vi "Car wash.vi"() -> ()   [LabVIEW 2019]
uses:
  <vilib>/regexp/Match Regular Expression.xnode
panel:
  out "STATE":string
  out "Vehicle Out Of Position":bool
  out "Air Dry LED":bool
  out "Clear Water Rinse":bool
  out "Main High Pressure Wash":bool
  out "Soap Application":bool
  out "Under Body Wash":bool
  out "Time Left (Sec)":dbl
  in  "Air Dry":bool
  in  "Main Wash":bool
  in  "Under Body":bool
  out "STOP":bool
  in  "stop":bool
  out "ECONOMY":bool
  out "DELUXE":bool
  in  "ECONOMY WASH":bool
  in  "DELUXE WASH":bool
  # "Car Wash Indicators"
  # "Under Body Wash"
  # "Soap Application"
  # "Main High Pressure Wash"
  # "Under Body Wash Position Switch"
  # "Clear Water Rinse"
  # "Main Wash Position Switch"
  # "Air Dry"
  # "Air Dry Position Switch"
  # "Vehicle Out of Position"
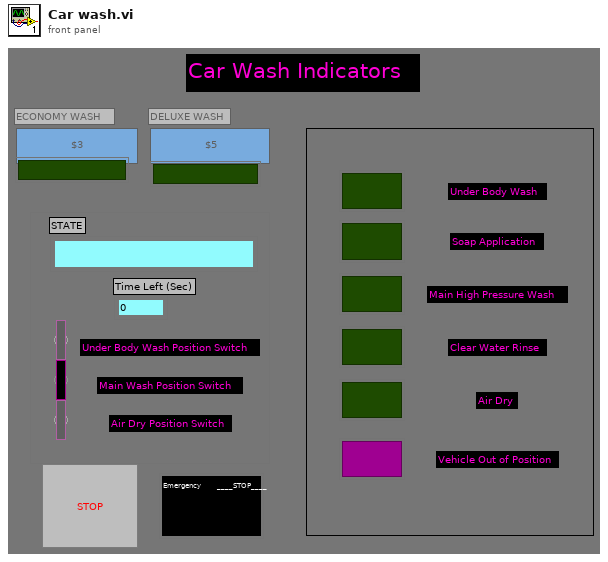
[diagram p1: front panel]
types:
  T1 = enum16{"Station", "Under Body", "Main Body", "Air Dry", "Report", "Stop"}
  T2 = enum8{"Enabled", "Disabled", "Disabled and Grayed Out"}
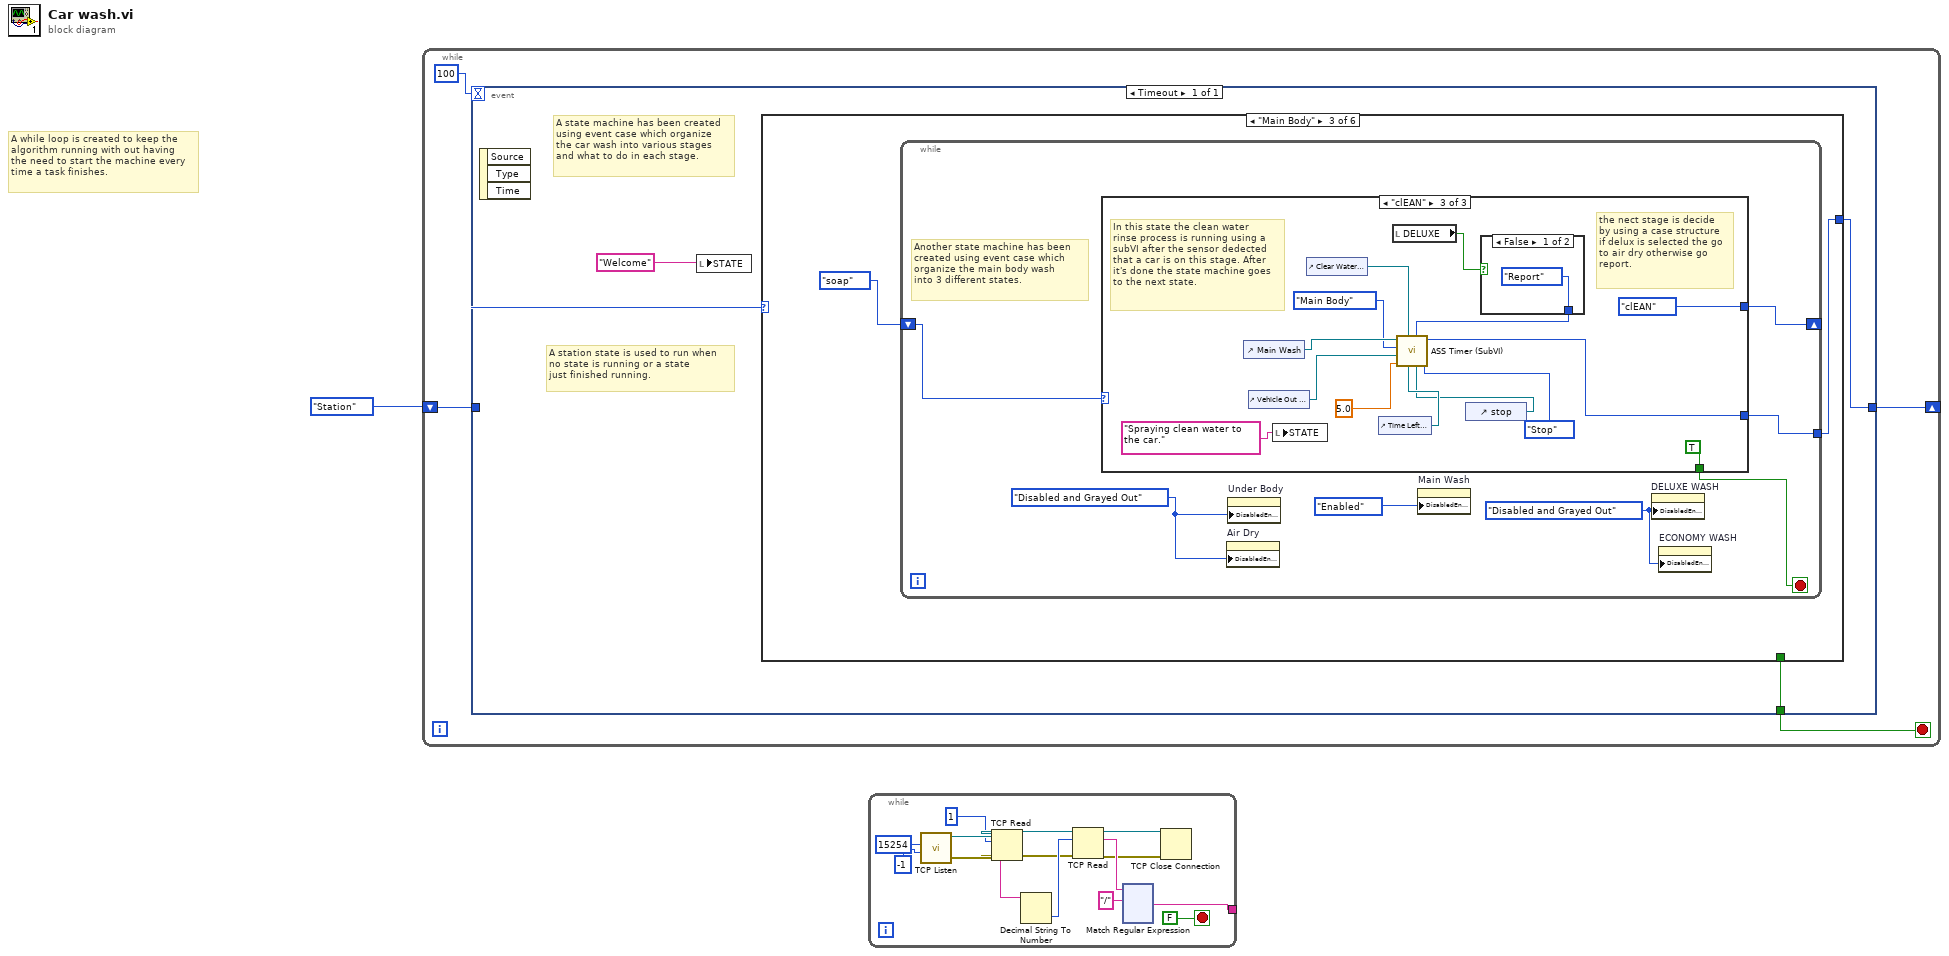
[diagram p0: block diagram]
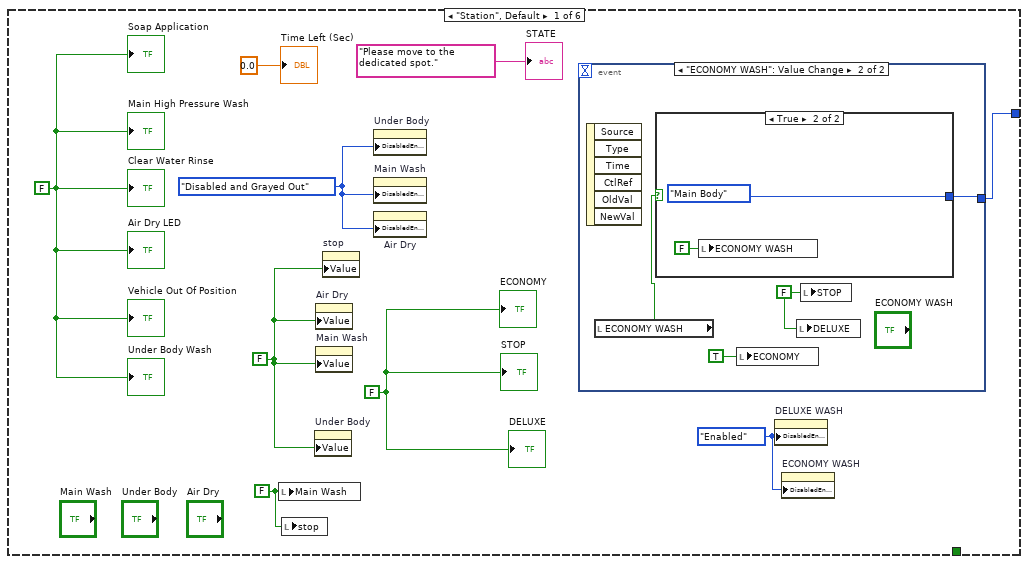
[diagram p2: hidden frame]
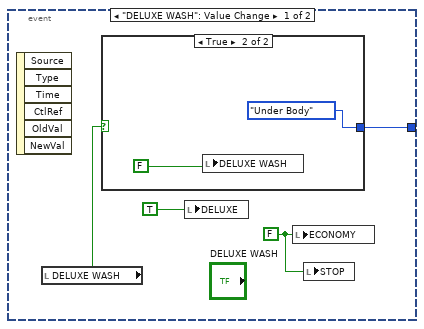
[diagram p3: hidden frame]
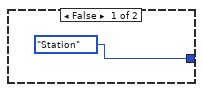
[diagram p4: hidden frame]
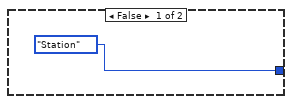
[diagram p5: hidden frame]
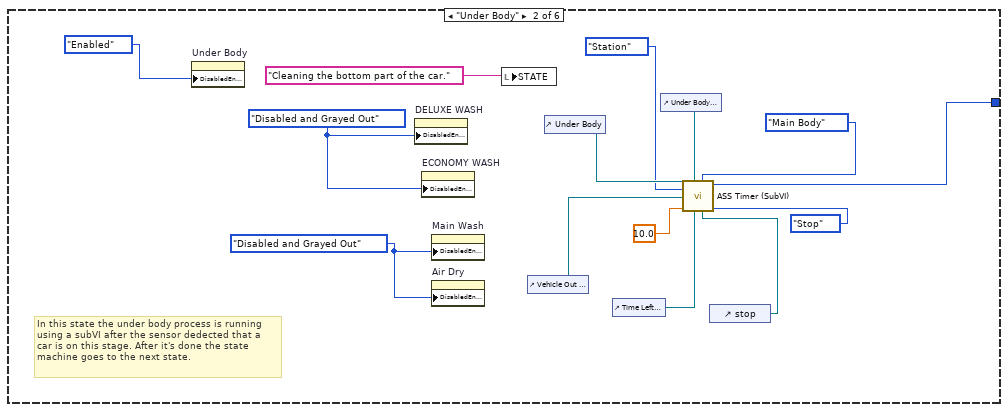
[diagram p6: hidden frame]
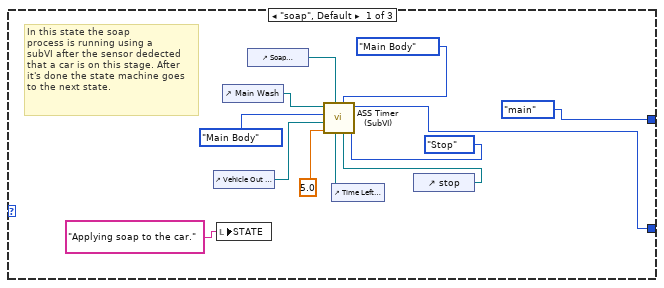
[diagram p7: hidden frame]
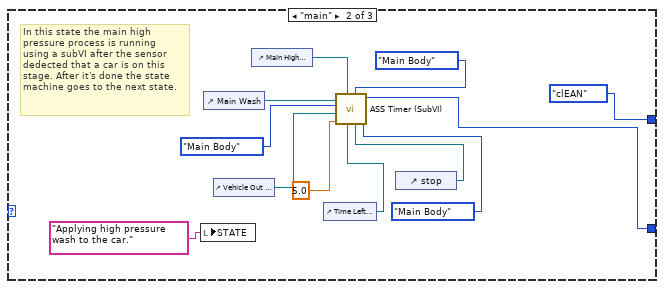
[diagram p8: hidden frame]
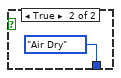
[diagram p9: hidden frame]
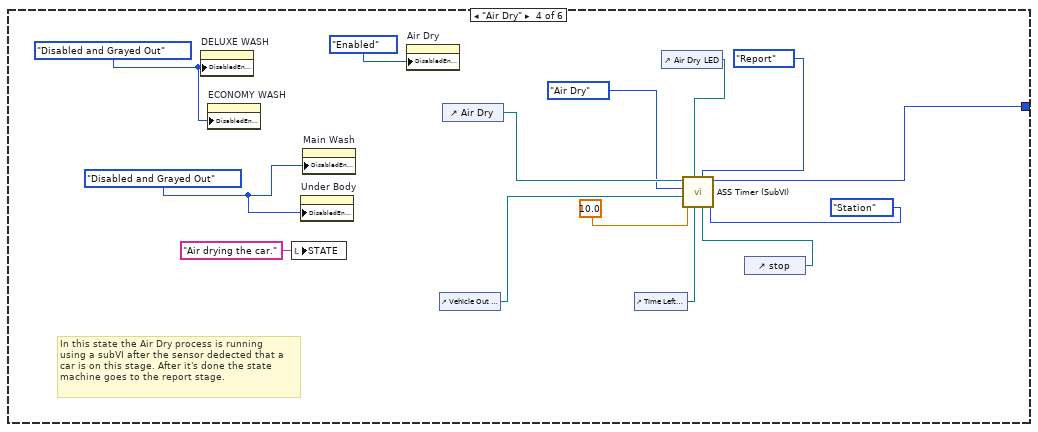
[diagram p10: hidden frame]
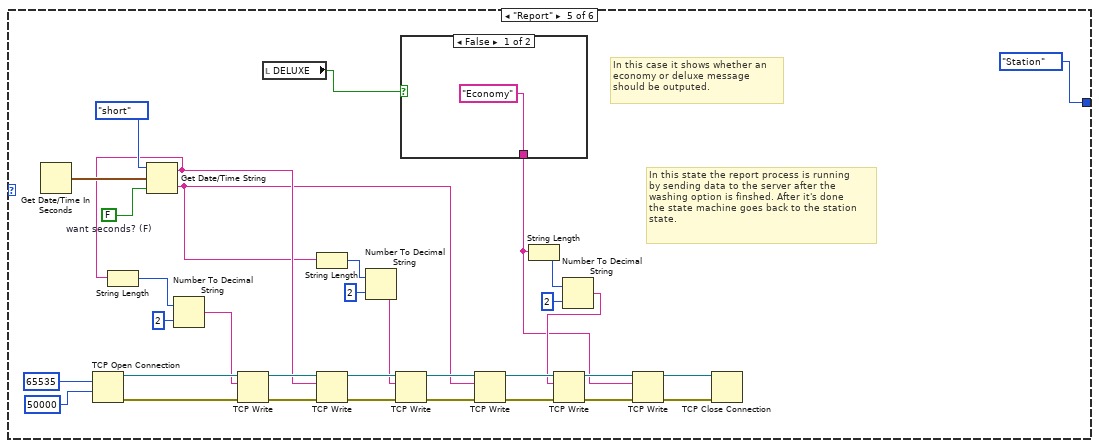
[diagram p11: hidden frame]
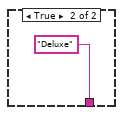
[diagram p12: hidden frame]
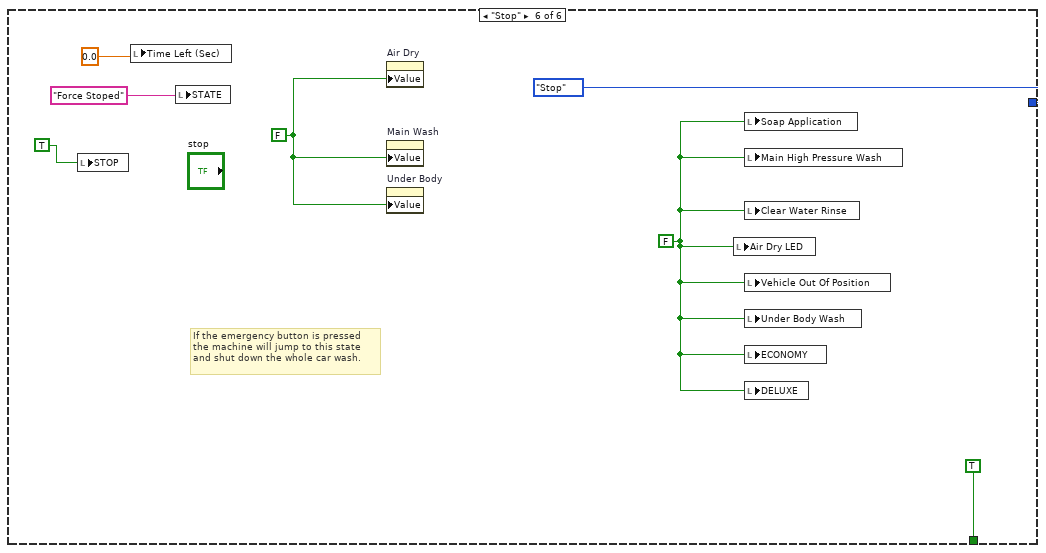
[diagram p13: hidden frame]
diagram:
  # "A while loop is created to keep the\nalgorithm running with out having\nthe need to start the machine every\ntime a task finishes."
  n1 = while {
    shift-right: [w3] -> _
    shift-left: T1."Station" -> [w4]
    stop <- w2 stop-if-true
    n2 = event shown="[0] Timeout" {
      selector: _ -> [_]
      dyn-events: _ -> [_]
      timeout: 100 -> [_]
      tunnel: w4 -> [w9]
      tunnel: [w8] -> w3
      tunnel: [w7] -> w2
      event Timeout {
        # "A station state is used to run when \nno state is running or a state \njust finished running."
        # "A state machine has been created\nusing event case which organize \nthe car wash into various stages \nand what to do in each stage."
        n3 = event-data() -> ()  [unwired: 1 in, 3 out]
        n4 = local write "STATE"("Welcome" ("STATE")) -> ()
        n5 = case shown="\"Main Body\"" w9 {
          tunnel: [w12 w33 w48 w109 T1."Station" T1."Stop"] -> w8
          tunnel: [_ _ _ _ _ TRUE] -> w7
          frame "Station", Default {
            w13 = T2."Enabled" ("Disabled")
            w14 = T2."Disabled and Grayed Out" ("Disabled")
            w15 = FALSE ("Main Wash")
            w17 = FALSE ("STOP")
            w10 = FALSE ("Vehicle Out")
            w18 = FALSE ("Clear Water Rinse")
            n6 = local write "Main Wash"(w15) -> ()
            n7 = local write "stop"(w15) -> ()
            n8 = property on="Under Body" class="Bool (strict)"("Value"=w10) -> ()  [unwired: 2 in, 2 out]
            n9 = property on="Air Dry" class="Bool (strict)"("Value"=w10) -> ()  [unwired: 2 in, 2 out]
            n10 = property on="Main Wash" class="Bool (strict)"("Value"=w10) -> ()  [unwired: 2 in, 2 out]
            n11 = property on="stop" class="Bool (strict)"("Value"=w10) -> ()  [unwired: 2 in, 2 out]
            n12 = property on="Under Body" class="Bool (strict)"("DisabledEnum"=w14) -> ()  [unwired: 2 in, 2 out]
            n13 = property on="Main Wash" class="Bool (strict)"("DisabledEnum"=w14) -> ()  [unwired: 2 in, 2 out]
            n14 = property on="Air Dry" class="Bool (strict)"("DisabledEnum"=w14) -> ()  [unwired: 2 in, 2 out]
            n15 = event shown="[1] \"ECONOMY WASH\": Value Change" {
              selector: _ -> [_ _]
              dyn-events: _ -> [_ _]
              timeout: _ -> [_ _]
              tunnel: [w19 w28] -> w12
              event "DELUXE WASH": Value Change {
                w20 = FALSE ("ECONOMY")
                n16 = event-data() -> ()  [unwired: 1 in, 6 out]
                n17 = local read "DELUXE WASH"() -> (w22:bool)
                n18 = case shown="True" w22 {
                  tunnel: [T1."Station" T1."Under Body"] -> w19
                  frame False {
                  }
                  frame True {
                    n19 = local write "DELUXE WASH"(FALSE ("ECONOMY WASH")) -> ()
                  }
                }
                n20 = local write "DELUXE"(TRUE ("DELUXE")) -> ()
                n21 = local write "ECONOMY"(w20) -> ()
                n22 = local write "STOP"(w20) -> ()
              }
              event "ECONOMY WASH": Value Change {
                w26 = FALSE ("STOP")
                n23 = event-data() -> ()  [unwired: 1 in, 6 out]
                n24 = local read "ECONOMY WASH"() -> (w29:bool)
                n25 = case shown="True" w29 {
                  tunnel: [T1."Station" T1."Main Body"] -> w28
                  frame False {
                  }
                  frame True {
                    n26 = local write "ECONOMY WASH"(FALSE ("ECONOMY WASH")) -> ()
                  }
                }
                n27 = local write "ECONOMY"(TRUE ("ECONOMY")) -> ()
                n28 = local write "DELUXE"(w26) -> ()
                n29 = local write "STOP"(w26) -> ()
              }
            }
            n30 = property on="DELUXE WASH" class="Bool (strict)"("DisabledEnum"=w13) -> ()  [unwired: 2 in, 2 out]
            n31 = property on="ECONOMY WASH" class="Bool (strict)"("DisabledEnum"=w13) -> ()  [unwired: 2 in, 2 out]
            "STATE" <- "Please move to the dedicated spot." ("STATE")
            "Soap Application" <- w18
            "Main High Pressure Wash" <- w18
            "Clear Water Rinse" <- w18
            "Air Dry LED" <- w18
            "Vehicle Out Of Position" <- w18
            "Under Body Wash" <- w18
            "DELUXE" <- w17
            "ECONOMY" <- w17
            "STOP" <- w17
            "Time Left (Sec)" <- 0.0 ("Time Left (Sec)")
          }
          frame "Under Body" {
            w41 = T2."Disabled and Grayed Out" ("Disabled")
            w40 = T2."Disabled and Grayed Out" ("Disabled")
            # "In this state the under body process is running\nusing a subVI after the sensor dedected that a\ncar is on this stage. After it's done the state\nmachine goes to the next state."
            n32 = property on="Under Body" class="Bool (strict)"("DisabledEnum"=T2."Enabled" ("Disabled")) -> ()  [unwired: 2 in, 2 out]
            n33 = property on="DELUXE WASH" class="Bool (strict)"("DisabledEnum"=w40) -> ()  [unwired: 2 in, 2 out]
            n34 = property on="ECONOMY WASH" class="Bool (strict)"("DisabledEnum"=w40) -> ()  [unwired: 2 in, 2 out]
            n35 = property on="Main Wash" class="Bool (strict)"("DisabledEnum"=w41) -> ()  [unwired: 2 in, 2 out]
            n36 = property on="Air Dry" class="Bool (strict)"("DisabledEnum"=w41) -> ()  [unwired: 2 in, 2 out]
            n37 = local write "STATE"("Cleaning the bottom part of the car." ("STATE")) -> ()
            n38 = control-ref of="Vehicle Out Of Position"() -> (w45:refnum<vi>)
            n39 = control-ref of="Under Body"() -> (w43:refnum<vi>)
            n40 = control-ref of="Time Left (Sec)"() -> (w44:refnum<vi>)
            n41 = control-ref of="Under Body Wash"() -> (w46:refnum<vi>)
            n42 = control-ref of="stop"() -> (w42:refnum<vi>)
            n43 = call "ASS Timer (SubVI).vi"("STOP Case"=T1."Stop", "STOP"=w42, "Next Case"=T1."Main Body", "Time"=w44, "Light"=w46, "Numeric"=10.0, "Vehicle Out Of Position"=w45, "Current Case"=T1."Station", "Switch"=w43) -> ("Case Out"=w33:T1)  [unwired: 2 in]
          }
          frame "Main Body" {
            n44 = while {
              shift-right: [w52] -> _
              shift-left: enum16{"soap", "main", "clEAN"}."soap" -> [w55]
              tunnel: [w53] -> w48
              stop <- w54 stop-if-true
              w49 = T2."Disabled and Grayed Out" ("Disabled")
              w50 = T2."Disabled and Grayed Out" ("Disabled")
              # "Another state machine has been \ncreated using event case which\norganize the main body wash \ninto 3 different states."
              n45 = case shown="\"clEAN\"" w55 {
                tunnel: [_ _ TRUE] -> w54
                tunnel: [w60 w73 w84] -> w53
                tunnel: [enum16{"soap", "main", "clEAN"}."main" enum16{"soap", "main", "clEAN"}."clEAN" enum16{"soap", "main", "clEAN"}."clEAN"] -> w52
                frame "soap", Default {
                  # "In this state the soap\nprocess is running using a \nsubVI after the sensor dedected\nthat a car is on this stage. After \nit's done the state machine goes\nto the next state."
                  n46 = control-ref of="Vehicle Out Of Position"() -> (w66:refnum<vi>)
                  n47 = local write "STATE"("Applying soap to the car." ("STATE")) -> ()
                  n48 = control-ref of="Main Wash"() -> (w67:refnum<vi>)
                  n49 = control-ref of="Soap Application"() -> (w62:refnum<vi>)
                  n50 = control-ref of="Time Left (Sec)"() -> (w64:refnum<vi>)
                  n51 = control-ref of="stop"() -> (w63:refnum<vi>)
                  n52 = call "ASS Timer (SubVI).vi"("STOP Case"=T1."Stop", "STOP"=w63, "Next Case"=T1."Main Body", "Time"=w64, "Light"=w62, "Numeric"=5.0, "Vehicle Out Of Position"=w66, "Current Case"=T1."Main Body", "Switch"=w67) -> ("Case Out"=w60:T1)  [unwired: 2 in]
                }
                frame "main" {
                  # "In this state the main high \npressure process is running \nusing a subVI after the sensor \ndedected that a car is on this \nstage. After it's done the state \nmachine goes to the next state."
                  n53 = local write "STATE"("Applying high pressure wash to the car." ("STATE")) -> ()
                  n54 = control-ref of="Main Wash"() -> (w79:refnum<vi>)
                  n55 = control-ref of="Vehicle Out Of Position"() -> (w78:refnum<vi>)
                  n56 = control-ref of="Main High Pressure Wash"() -> (w74:refnum<vi>)
                  n57 = control-ref of="Time Left (Sec)"() -> (w76:refnum<vi>)
                  n58 = control-ref of="stop"() -> (w75:refnum<vi>)
                  n59 = call "ASS Timer (SubVI).vi"("STOP Case"=T1."Main Body", "STOP"=w75, "Next Case"=T1."Main Body", "Time"=w76, "Light"=w74, "Numeric"=5.0, "Vehicle Out Of Position"=w78, "Current Case"=T1."Main Body", "Switch"=w79) -> ("Case Out"=w73:T1)  [unwired: 2 in]
                }
                frame "clEAN" {
                  # "the nect stage is decide\nby using a case structure\nif delux is selected the go\nto air dry otherwise go \nreport."
                  # "In this state the clean water\nrinse process is running using a \nsubVI after the sensor dedected\nthat a car is on this stage. After \nit's done the state machine goes\nto the next state."
                  n60 = control-ref of="Main Wash"() -> (w92:refnum<vi>)
                  n61 = control-ref of="Vehicle Out Of Position"() -> (w91:refnum<vi>)
                  n62 = local write "STATE"("Spraying clean water to the car." ("STATE")) -> ()
                  n63 = control-ref of="Clear Water Rinse"() -> (w88:refnum<vi>)
                  n64 = control-ref of="Time Left (Sec)"() -> (w90:refnum<vi>)
                  n65 = local read "DELUXE"() -> (w83:bool)
                  n66 = control-ref of="stop"() -> (w89:refnum<vi>)
                  n67 = case shown="False" w83 {
                    tunnel: [T1."Report" T1."Air Dry"] -> w87
                    frame False {
                    }
                    frame True {
                    }
                  }
                  n68 = call "ASS Timer (SubVI).vi"("STOP Case"=T1."Stop", "STOP"=w89, "Next Case"=w87, "Time"=w90, "Light"=w88, "Numeric"=5.0, "Vehicle Out Of Position"=w91, "Current Case"=T1."Main Body", "Switch"=w92) -> ("Case Out"=w84:T1)  [unwired: 2 in]
                }
              }
              n69 = property on="Air Dry" class="Bool (strict)"("DisabledEnum"=w50) -> ()  [unwired: 2 in, 2 out]
              n70 = property on="Under Body" class="Bool (strict)"("DisabledEnum"=w50) -> ()  [unwired: 2 in, 2 out]
              n71 = property on="Main Wash" class="Bool (strict)"("DisabledEnum"=T2."Enabled" ("Disabled")) -> ()  [unwired: 2 in, 2 out]
              n72 = property on="DELUXE WASH" class="Bool (strict)"("DisabledEnum"=w49) -> ()  [unwired: 2 in, 2 out]
              n73 = property on="ECONOMY WASH" class="Bool (strict)"("DisabledEnum"=w49) -> ()  [unwired: 2 in, 2 out]
            }
          }
          frame "Air Dry" {
            w99 = T2."Disabled and Grayed Out" ("Disabled")
            w101 = T2."Disabled and Grayed Out" ("Disabled")
            # "In this state the Air Dry process is running\nusing a subVI after the sensor dedected that a\ncar is on this stage. After it's done the state\nmachine goes to the report stage."
            n74 = property on="DELUXE WASH" class="Bool (strict)"("DisabledEnum"=w99) -> ()  [unwired: 2 in, 2 out]
            n75 = property on="ECONOMY WASH" class="Bool (strict)"("DisabledEnum"=w99) -> ()  [unwired: 2 in, 2 out]
            n76 = local write "STATE"("Air drying the car." ("STATE")) -> ()
            n77 = property on="Under Body" class="Bool (strict)"("DisabledEnum"=w101) -> ()  [unwired: 2 in, 2 out]
            n78 = property on="Main Wash" class="Bool (strict)"("DisabledEnum"=w101) -> ()  [unwired: 2 in, 2 out]
            n79 = property on="Air Dry" class="Bool (strict)"("DisabledEnum"=T2."Enabled" ("Disabled")) -> ()  [unwired: 2 in, 2 out]
            n80 = control-ref of="Vehicle Out Of Position"() -> (w106:refnum<vi>)
            n81 = control-ref of="Air Dry"() -> (w104:refnum<vi>)
            n82 = control-ref of="Time Left (Sec)"() -> (w107:refnum<vi>)
            n83 = control-ref of="Air Dry LED"() -> (w105:refnum<vi>)
            n84 = control-ref of="stop"() -> (w103:refnum<vi>)
            n85 = call "ASS Timer (SubVI).vi"("STOP Case"=T1."Station", "STOP"=w103, "Next Case"=T1."Report", "Time"=w107, "Light"=w105, "Numeric"=10.0, "Vehicle Out Of Position"=w106, "Current Case"=T1."Air Dry", "Switch"=w104) -> ("Case Out"=w109:T1)  [unwired: 2 in]
          }
          frame "Report" {
            w132 = FALSE  # want seconds? (F)
            # "In this case it shows whether an \neconomy or deluxe message \nshould be outputed."
            # "In this state the report process is running\nby sending data to the server after the \nwashing option is finshed. After it's done \nthe state machine goes back to the station \nstate."
            n86 = Get Date/Time In Seconds() -> (seconds since 1Jan1904=w133:timestamp)
            n87 = TCP Open Connection(remote port or service name=u16 65535, timeout ms (60000)=50000) -> (connection ID=w138:refnum<k5>, error out=w141:errorcluster)  [unwired: 3 in]
            n88 = Get Date/Time String(date format (0)=enum16{"short", "long", "abbreviated"}."short", seconds (now)=w133, want seconds? (F)=w132) -> (date string=w121:string, time string=w118:string)
            n89 = String Length(string=w121) -> (length=w123:i32)
            n90 = Number To Decimal String(number=w123, width (-)=i16 2) -> (decimal integer string=w122:string)
            n91 = TCP Write(connection ID=w138, data in=w122, error in (no error)=w141) -> (connection ID out=w137:refnum<k5>, error out=w140:errorcluster)  [unwired: 1 in, 1 out]
            n92 = local read "DELUXE"() -> (w117:bool)
            n93 = String Length(string=w118) -> (length=w120:i32)
            n94 = TCP Write(connection ID=w137, data in=w121, error in (no error)=w140) -> (connection ID out=w136:refnum<k5>, error out=w139:errorcluster)  [unwired: 1 in, 1 out]
            n95 = Number To Decimal String(number=w120, width (-)=i16 2) -> (decimal integer string=w119:string)
            n96 = TCP Write(connection ID=w136, data in=w119, error in (no error)=w139) -> (connection ID out=w131:refnum<k5>, error out=w130:errorcluster)  [unwired: 1 in, 1 out]
            n97 = case shown="False" w117 {
              tunnel: ["Economy" "Deluxe"] -> w114
              frame False {
              }
              frame True {
              }
            }
            n98 = TCP Write(connection ID=w131, data in=w118, error in (no error)=w130) -> (connection ID out=w128:refnum<k5>, error out=w124:errorcluster)  [unwired: 1 in, 1 out]
            n99 = String Length(string=w114) -> (length=w116:i32)
            n100 = Number To Decimal String(number=w116, width (-)=i16 2) -> (decimal integer string=w115:string)
            n101 = TCP Write(connection ID=w128, data in=w115, error in (no error)=w124) -> (connection ID out=w127:refnum<k5>, error out=w129:errorcluster)  [unwired: 1 in, 1 out]
            n102 = TCP Write(connection ID=w127, data in=w114, error in (no error)=w129) -> (connection ID out=w126:refnum<k5>, error out=w125:errorcluster)  [unwired: 1 in, 1 out]
            n103 = TCP Close Connection(connection ID=w126, error in (no error)=w125) -> ()  [unwired: 1 in, 2 out]
          }
          frame "Stop" {
            w149 = FALSE ("Air Dry")
            w148 = FALSE ("Vehicle Out")
            # "If the emergency button is pressed\nthe machine will jump to this state\nand shut down the whole car wash."
            n104 = local write "STOP"(TRUE ("STOP")) -> ()
            n105 = local write "Time Left (Sec)"(0.0 ("Time Left (Sec)")) -> ()
            n106 = local write "STATE"("Force Stoped" ("STATE")) -> ()
            n107 = property on="Air Dry" class="Bool (strict)"("Value"=w148) -> ()  [unwired: 2 in, 2 out]
            n108 = property on="Main Wash" class="Bool (strict)"("Value"=w148) -> ()  [unwired: 2 in, 2 out]
            n109 = property on="Under Body" class="Bool (strict)"("Value"=w148) -> ()  [unwired: 2 in, 2 out]
            n110 = local write "Air Dry LED"(w149) -> ()
            n111 = local write "Soap Application"(w149) -> ()
            n112 = local write "Main High Pressure Wash"(w149) -> ()
            n113 = local write "Clear Water Rinse"(w149) -> ()
            n114 = local write "Vehicle Out Of Position"(w149) -> ()
            n115 = local write "Under Body Wash"(w149) -> ()
            n116 = local write "ECONOMY"(w149) -> ()
            n117 = local write "DELUXE"(w149) -> ()
          }
        }
      }
    }
  }
  n118 = while {
    tunnel: [w152] -> _
    stop <- FALSE stop-if-true
    n119 = call <vilib>:"TCP Listen.vi"("timeout ms (wait forever: -1)"=-1, "port"=u16 15254) -> ("error out"=w163:errorcluster, "connection ID"=w158:refnum<k5>)  [unwired: 5 in, 3 out]
    n120 = TCP Read(connection ID=w158, bytes to read=1, error in (no error)=w163) -> (connection ID out=w159:refnum<k5>, data out=w164:string, error out=w162:errorcluster)  [unwired: 2 in]
    n121 = Decimal String To Number(string=w164) -> (number=w165:i32)  [unwired: 2 in, 1 out]
    n122 = TCP Read(connection ID=w159, bytes to read=w165, error in (no error)=w162) -> (connection ID out=w160:refnum<k5>, data out=w166:string, error out=w161:errorcluster)  [unwired: 2 in]
    n123 = xnode "Match Regular Expression"("input string"=w166, "regular expression"="/") -> ("after match"=w152:string)  [unwired: 4 in, 4 out]
    n124 = TCP Close Connection(connection ID=w160, error in (no error)=w161) -> ()  [unwired: 1 in, 2 out]
  }
